vi "iHR550 Set Values v10.5.0.vi"(0 "Refnum out":refnum<k7>, 1 "Entrance Mirror":u16(ring)=2 caption="Target Position\nEntrance Mirror" items=["Front"=2, "Side"=3], 3 "Target\nSide Entrance":dbl, 5 "iHR Settings":T1={"iHR550 Set Exit Mirror"=2, "iHR550 Set Side Exit"=0.0, "iHR550 Set Front Entrance"=0.0, "iHR550 Set Wavelength"=897.9988, "iHR550 Set Grating"=0, "iHR550 Set Grating Switch"=FALSE, "iHR550 Set Wavelength Switch"=FALSE, "iHR550 Set Mirror Switch"=FALSE, "iHR550 Set Slits Switch"=FALSE} {"iHR550 Set Wavelength" min=0.0 max=1500.0 step=1.0; "iHR550 Set Side Exit" min=0.0 max=2000.0 step=1.0; "iHR550 Set Exit Mirror" items=["Front"=2, "Side"=3]}, 11 "error in (no error)":errorcluster, 13 "Target\nFront Exit":dbl) -> (15 "error out":errorcluster)   [LabVIEW 2010]
uses:
  TypeDefs/iHR Settings.ctl
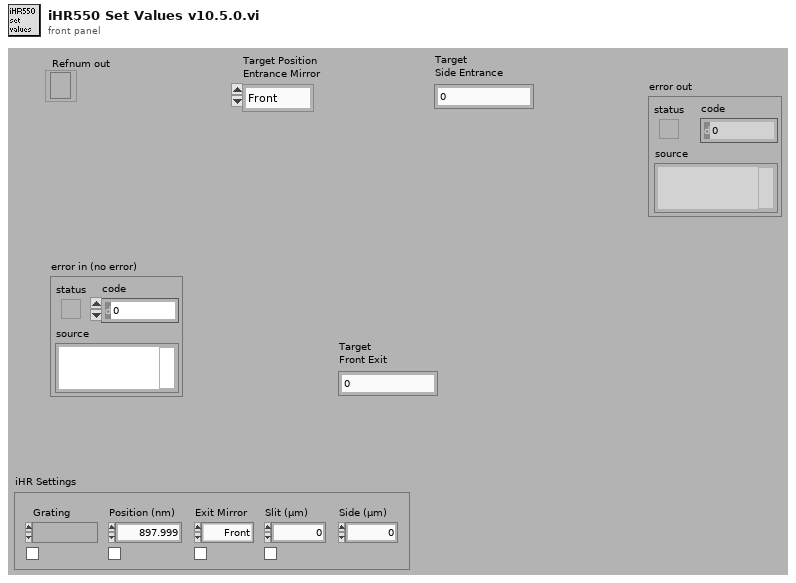
[diagram p1: front panel]
types:
  T1 = typedef "iHR Settings.ctl" = cluster{"iHR550 Set Exit Mirror":u16, "iHR550 Set Side Exit":dbl, "iHR550 Set Front Entrance":dbl, "iHR550 Set Wavelength":dbl, "iHR550 Set Grating":u16, "iHR550 Set Grating Switch":bool, "iHR550 Set Wavelength Switch":bool, "iHR550 Set Mirror Switch":bool, "iHR550 Set Slits Switch":bool}
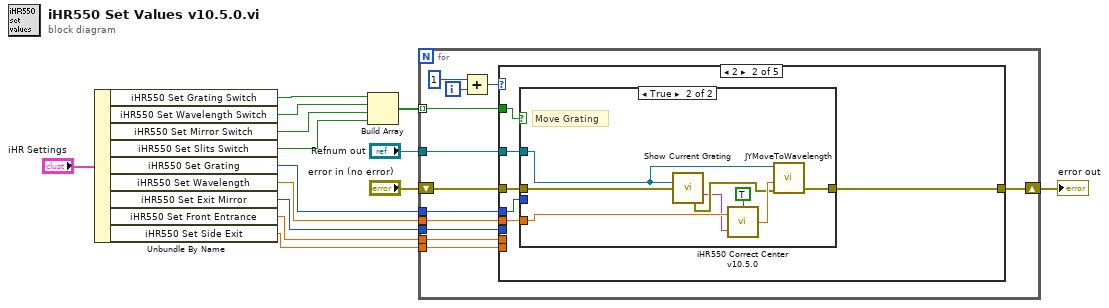
[diagram p0: block diagram]
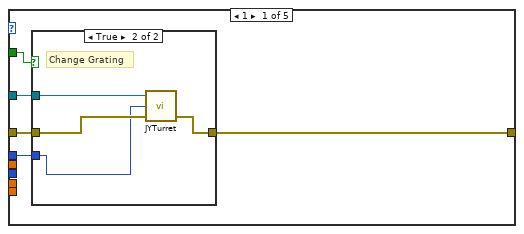
[diagram p2: hidden frame]
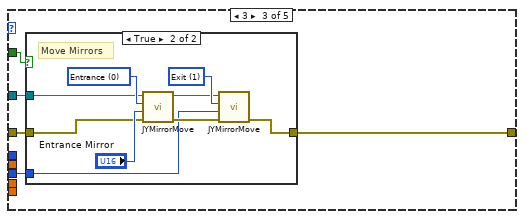
[diagram p5: hidden frame]
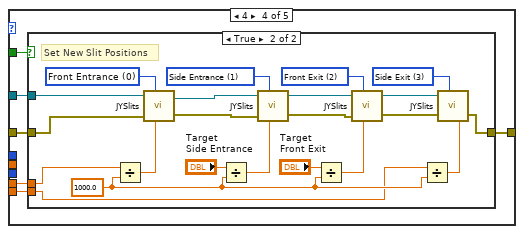
[diagram p7: hidden frame]
diagram:
  n1 = Unbundle By Name("iHR Settings") -> ("iHR550 Set Grating Switch"=w7:bool, "iHR550 Set Wavelength Switch"=w10:bool, "iHR550 Set Mirror Switch"=w9:bool, "iHR550 Set Slits Switch"=w8:bool, "iHR550 Set Grating"=w5:u16, "iHR550 Set Wavelength"=w4:dbl, "iHR550 Set Exit Mirror"=w3:u16, "iHR550 Set Front Entrance"=w2:dbl, "iHR550 Set Side Exit"=w1:dbl)
  n2 = Build Array(w7, w10, w9, w8) -> (w6:bool[])
  n3 = for {
    tunnel: w6 -> [w26] mode=indexing
    tunnel: "Refnum out" -> [w25]
    shift-right: [w24] -> w13
    shift-left: "error in (no error)" -> [w23]
    tunnel: w5 -> [w19]
    tunnel: w4 -> [w18]
    tunnel: w3 -> [w17]
    tunnel: w2 -> [w16]
    tunnel: w1 -> [w15]
    i -> [w22]
    n4 = Add(x=1, y=w22) -> (x+y=w20:i32)
    n5 = case shown="2" w20 {
      tunnel: w26 -> [w31 w39 w53 w72 _]
      tunnel: w25 -> [w30 w40 w54 w69 _]
      tunnel: [w29 w42 w55 w70 w96] -> w24
      tunnel: w23 -> [w28 w41 w56 w71 w96]
      tunnel: w19 -> [w27 w37 _ _ _]
      tunnel: w18 -> [_ w38 _ _ _]
      tunnel: w17 -> [_ _ w52 _ _]
      tunnel: w16 -> [_ _ _ w68 _]
      tunnel: w15 -> [_ _ _ w67 _]
      frame 1 {
        n6 = case shown="True" w31 {
          tunnel: w30 -> [_ w36]
          tunnel: [w32 w35] -> w29
          tunnel: w28 -> [w32 w34]
          tunnel: w27 -> [_ w33]
          frame False {
          }
          frame True {
            # "Change Grating"
            n7 = call "JYTurret.vi"("error in (no error)"=w34, "Grating Index"=w33, "JYMONOLib.IJYMonoReqd"=w36) -> ("error out"=w35:errorcluster)  [unwired: 2 out]
          }
        }
      }
      frame 2 {
        n8 = case shown="True" w39 {
          tunnel: w40 -> [_ w45]
          tunnel: w41 -> [w43 w47]
          tunnel: [w43 w51] -> w42
          tunnel: w38 -> [_ w50]
          tunnel: w37 -> [_ _]
          frame False {
          }
          frame True {
            # "Move Grating"
            n9 = call "Show Current Grating.vi"("Refnum in"=w45, "error in (no error)"=w47) -> ("Current Description"=w44:string, "error out"=w46:errorcluster)  [unwired: 5 in, 7 out]
            n10 = call "iHR550 Correct Center v10.5.0.vi"("Set?"=TRUE, "Description"=w44, "Position In (nm)"=w50) -> ("Position Out (nm)"=w48:dbl)
            n11 = call "JYMoveToWavelength.vi"("error in (no error)"=w46, "Target WL"=w48, "RefNum In"=w45) -> ("error out"=w51:errorcluster)  [unwired: 1 in, 2 out]
          }
        }
      }
      frame 3 {
        n12 = case shown="True" w53 {
          tunnel: w56 -> [w57 w62]
          tunnel: [w57 w61] -> w55
          tunnel: w54 -> [_ w59]
          tunnel: w52 -> [_ w60]
          frame False {
          }
          frame True {
            w65 = u16 1 items=["Entrance", "Exit", "Front", "Side"] ("Mirror Number")
            w63 = u16 0 items=["Entrance", "Exit", "Front", "Side"] ("Mirror Number")
            # "Move Mirrors"
            n13 = call "JYMirrorMove.vi"("error in (no error)"=w62, "Mirror Position"="Entrance Mirror", "Mirror Number"=w63, "RefNum In"=w59) -> ("error out"=w66:errorcluster, "MonoRefNum Out"=w58:refnum<k7>)  [unwired: 6 in]
            n14 = call "JYMirrorMove.vi"("error in (no error)"=w66, "Mirror Position"=w60, "Mirror Number"=w65, "RefNum In"=w58) -> ("error out"=w61:errorcluster)  [unwired: 6 in, 1 out]
          }
        }
      }
      frame 4 {
        n15 = case shown="True" w72 {
          tunnel: w71 -> [w73 w85]
          tunnel: [w73 w83] -> w70
          tunnel: w69 -> [_ w84]
          tunnel: w68 -> [_ w75]
          tunnel: w67 -> [_ w74]
          frame False {
          }
          frame True {
            w82 = 1000.0 ("y")
            w95 = u16 3 items=["Front Entrance", "Side Entrance", "Front Exit", "Side Exit", "First Intermediate", "Second Intermediate"] ("Slit")
            w94 = u16 2 items=["Front Entrance", "Side Entrance", "Front Exit", "Side Exit", "First Intermediate", "Second Intermediate"] ("Slit")
            w93 = u16 1 items=["Front Entrance", "Side Entrance", "Front Exit", "Side Exit", "First Intermediate", "Second Intermediate"] ("Slit")
            w92 = u16 0 items=["Front Entrance", "Side Entrance", "Front Exit", "Side Exit", "First Intermediate", "Second Intermediate"] ("Slit")
            # "Set New Slit Positions"
            n16 = Divide(x=w75, y=w82) -> (x/y=w79:dbl)
            n17 = call "JYSlits.vi"("JYMONOLib.IJYMonoReqd"=w84, "Slit"=w92, "error in (no error)"=w85, "Slit Width"=w79) -> ("JYMONOLib.IJYMonoReqd 2"=w86:refnum<k7>, "error out"=w89:errorcluster)  [unwired: 1 in]
            n18 = Divide(x="Target\nSide Entrance", y=w82) -> (x/y=w78:dbl)
            n19 = call "JYSlits.vi"("JYMONOLib.IJYMonoReqd"=w86, "Slit"=w93, "error in (no error)"=w89, "Slit Width"=w78) -> ("JYMONOLib.IJYMonoReqd 2"=w87:refnum<k7>, "error out"=w90:errorcluster)  [unwired: 1 in]
            n20 = Divide(x="Target\nFront Exit", y=w82) -> (x/y=w77:dbl)
            n21 = call "JYSlits.vi"("JYMONOLib.IJYMonoReqd"=w87, "Slit"=w94, "error in (no error)"=w90, "Slit Width"=w77) -> ("JYMONOLib.IJYMonoReqd 2"=w88:refnum<k7>, "error out"=w91:errorcluster)  [unwired: 1 in]
            n22 = Divide(x=w74, y=w82) -> (x/y=w76:dbl)
            n23 = call "JYSlits.vi"("JYMONOLib.IJYMonoReqd"=w88, "Slit"=w95, "error in (no error)"=w91, "Slit Width"=w76) -> ("error out"=w83:errorcluster)  [unwired: 1 in, 1 out]
          }
        }
      }
      frame 5, Default {
      }
    }
  }
  "error out" <- w13
